vi "clear all input channels.vi"(10 "engine configuration in":refnum<class "engine configuration.lvclass">, 11 "TEC configuration in":refnum<class "TEC configuration.lvclass">) -> (2 "engine configuration out":refnum<class "engine configuration.lvclass">, 3 "TEC configuration out":refnum<class "TEC configuration.lvclass">)   [LabVIEW 2013, in "TEC editor node.lvclass"]
uses:
  TEC editor node.lvclass
  configuration/TEC configuration.lvclass
  <vilib>/NI/Module Execution Interface/Engine Configuration/engine configuration.lvclass
  <vilib>/NI/Tag Bus Module Framework/channel/channel classification.ctl
  <vilib>/NI/Configuration Framework/serializable configuration/NISE_CEF_serializable configuration.lvclass/NISE_CEF_serializable configuration.ctl
  <vilib>/NI/Configuration Framework/serializable configuration/NISE_CEF_serializable configuration.lvclass
  <vilib>/NI/Tag Bus/tag/tag descriptor.lvclass/tag descriptor.ctl
  <vilib>/NI/Tag Bus Module Framework/channel/TBM channel.lvclass
  <vilib>/NI/Tag Bus/tag/tag descriptor.lvclass
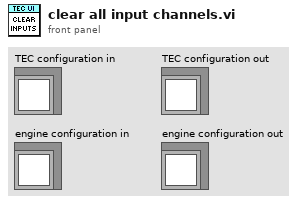
[diagram p1: front panel]
types:
  T1 = typedef "TBM channel.lvclass/channel classification.ctl" = enum16{"input data", "output data", "processing parameter", "processing result"}
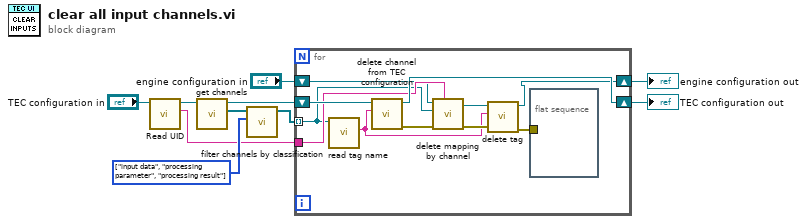
[diagram p0: block diagram]
diagram:
  w7 = T1[] [enum."input data", enum."processing parameter", enum."processing result"] items=["input data", "output data", "processing parameter", "processing result"] ("allowed classifications")
  n1 = call <vilib>:"Read UID.vi"("configuration in"="TEC configuration in") -> ("instance id"=w3:string, "configuration out"=w4:refnum<class "TEC configuration.lvclass">)  [unwired: 8 in, 1 out]
  n2 = call-dynamic "get channels.vi"("TEC configuration in"=w4) -> ("channels"=w8:refnum<class "TBM channel.lvclass">[], "TEC configuration out"=w6:refnum<class "TEC configuration.lvclass">)  [unwired: 9 in]
  n3 = call <vilib>:"filter channels by classification.vi"("allowed classifications"=w7, "channels in"=w8) -> ("channels out"=w9:refnum<class "TBM channel.lvclass">[])  [unwired: 9 in]
  n4 = for {
    shift-right: [w20] -> w10
    shift-left: w6 -> [w21]
    tunnel: w9 -> [w16] mode=indexing
    tunnel: w3 -> [w19]
    shift-right: [w12] -> w1
    shift-left: "engine configuration in" -> [w18]
    n5 = call <vilib>:"read tag name.vi"("system tag in"=w16) -> ("name"=w11:string)  [unwired: 8 in, 2 out]
    n6 = call "delete channel from TEC configuration.vi"("channel to delete"=w11, "TEC configuration in"=w21) -> ("error out"=w17:errorcluster, "TEC configuration out"=w20:refnum<class "TEC configuration.lvclass">)  [unwired: 8 in]
    n7 = call <vilib>:"delete mapping by channel.vi"("owner ID"=w19, "error in"=w17, "channel"=w16, "engine configuration in"=w18) -> ("error out"=w14:errorcluster, "engine configuration out"=w15:refnum<class "engine configuration.lvclass">)  [unwired: 6 in]
    n8 = call <vilib>:"delete tag.vi"("error in"=w14, "tag name"=w11, "engine configuration in"=w15) -> ("error out"=w13:errorcluster, "engine configuration out"=w12:refnum<class "engine configuration.lvclass">)  [unwired: 7 in]
    n9 = flat-sequence {
      tunnel: w13 -> [_]
      frame #0 {
      }
    }
  }
  "TEC configuration out" <- w10
  "engine configuration out" <- w1
